vi "Get Terminal Refs for New Frame.vi"(8 "error in (no error)":errorcluster, 10 "Case Structure Ref":refnum<vi>, 11 "Setter Generator In":refnum<class "Setter Generator.lvclass">) -> (0 "error out":errorcluster, 2 "reference out":refnum<vi>, 3 "Setter Generator Out":refnum<class "Setter Generator.lvclass">)   [LabVIEW 2020, in "Method Generation.lvlib" / "Setter Generator.lvclass"]
uses:
  Setter Generator.lvclass
  Setter Generator.lvclass/Setter Generator.ctl
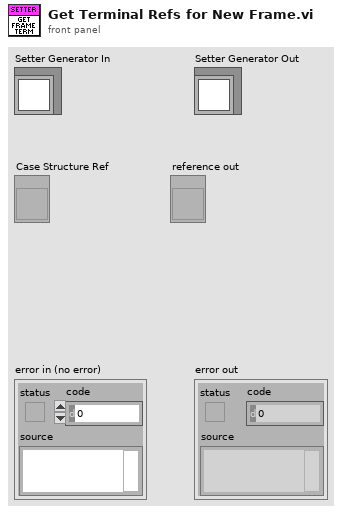
[diagram p1: front panel]
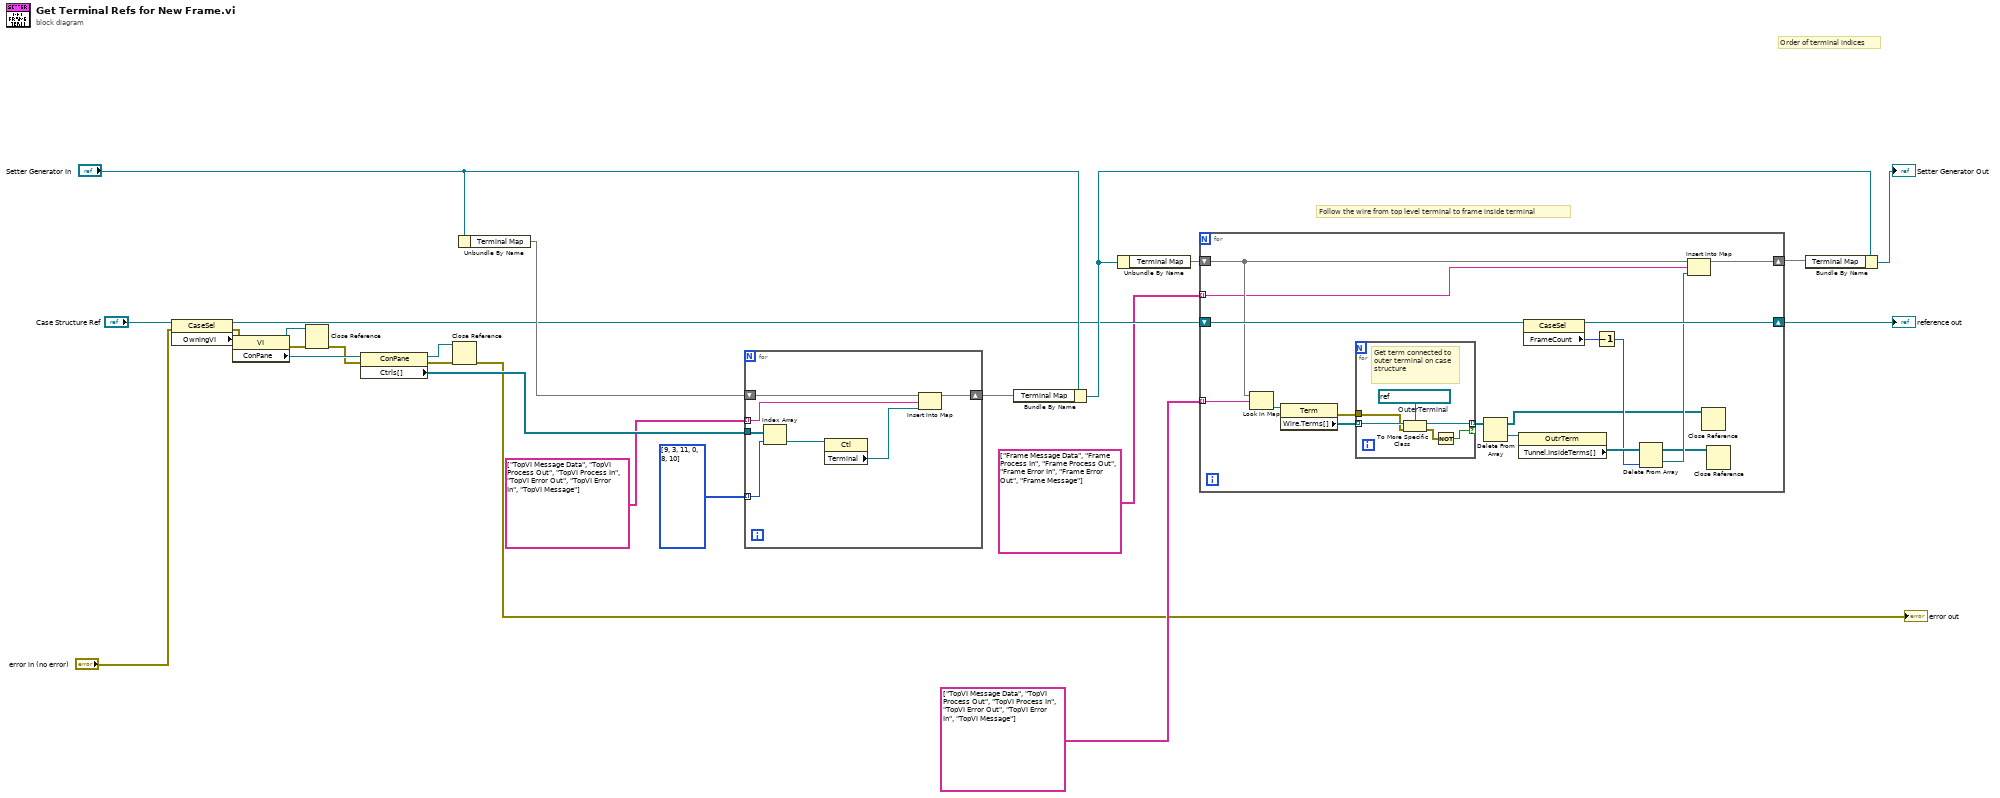
[diagram p0: block diagram]
diagram:
  # "Follow the wire from top level terminal to frame inside terminal"
  # "Order of terminal indices"
  n1 = property class="CaseSel"(reference="Case Structure Ref", error in="error in (no error)") -> (reference out=w15:refnum<vi>, error out=w19:errorcluster, "OwningVI"=w25:refnum<vi>)
  n2 = property class="VI"(reference=w25, error in=w19) -> (reference out=w7:refnum<vi>, error out=w18:errorcluster, "ConPane"=w23:refnum<vi>)
  n3 = Close Reference(reference=w7, error in (no error)=w18) -> (error out=w8:errorcluster)
  n4 = property class="ConPane"(reference=w23, error in=w8) -> (reference out=w5:refnum<vi>, error out=w6:errorcluster, "Ctrls[]"=w24:refnum<vi>[])
  n5 = Close Reference(reference=w5, error in (no error)=w6) -> (error out=→"error out":errorcluster)
  n6 = Unbundle By Name("Setter Generator In") -> ("Terminal Map"=w20:map{string, refnum<vi>})
  n7 = for {
    tunnel: w24 -> [w30]
    shift-right: [w31] -> w10
    shift-left: w20 -> [w32]
    tunnel: i32[] [9, 3, 11, 0, 8, 10] ("index") -> [w29] mode=indexing
    tunnel: string[] ["TopVI Message Data", "TopVI Process Out", "TopVI Process In", "TopVI Error Out", "TopVI Error In", "TopVI Message"] ("Array") -> [w26] mode=indexing
    n8 = Index Array(array=w30, index=w29) -> (element=w28:refnum<vi>)
    n9 = property class="Ctl"(reference=w28) -> ("Terminal"=w27:refnum<vi>)  [unwired: 1 in, 2 out]
    n10 = Insert Into Map(map in=w32, key=w26, value=w27) -> (map out=w31:map{string, refnum<vi>})  [unwired: 2 out]
  }
  n11 = Bundle By Name(cluster="Setter Generator In", "Terminal Map"=w10) -> (w16:refnum<class "Setter Generator.lvclass">)
  n12 = Unbundle By Name(w16) -> ("Terminal Map"=w13:map{string, refnum<vi>})
  n13 = for {
    shift-right: [w40] -> w14
    shift-left: w15 -> [w43]
    shift-right: [w36] -> w11
    shift-left: w13 -> [w39]
    tunnel: string[] ["TopVI Message Data", "TopVI Process Out", "TopVI Process In", "TopVI Error Out", "TopVI Error In", "TopVI Message"] ("Array") -> [w38] mode=indexing
    tunnel: string[] ["Frame Message Data", "Frame Process In", "Frame Process Out", "Frame Error In", "Frame Error Out", "Frame Message"] -> [w37] mode=indexing
    n14 = Look In Map(map=w39, key=w38) -> (value=w49:refnum<vi>)  [unwired: 1 in, 1 out]
    n15 = property class="Term"(reference=w49) -> (error out=w47:errorcluster, "Wire.Terms[]"=w48:refnum<vi>[])  [unwired: 1 in, 1 out]
    n16 = for {
      tunnel: w48 -> [w55] mode=indexing
      tunnel: [w53] -> w46 mode=indexing if=w51
      tunnel: w47 -> [w50]
      w54 = refnum<vi> refnum  # OuterTerminal
      # "Get term connected to outer terminal on case structure"
      n17 = To More Specific Class(target class=w54, reference=w55, error in=w50) -> (specific class reference=w53:refnum<vi>, error out=w52:errorcluster)
      n18 = Not(x=w52) -> (.not. x?=w51:bool)
    }
    n19 = Delete From Array(array=w46) -> (deleted portion=w45:refnum<vi>, array with subset deleted=w33:refnum<vi>[])  [unwired: 2 in]
    n20 = property class="OutrTerm"(reference=w45) -> ("Tunnel.InsideTerms[]"=w44:refnum<vi>[])  [unwired: 1 in, 2 out]
    n21 = property class="CaseSel"(reference=w43) -> (reference out=w40:refnum<vi>, "FrameCount"=w42:i32)  [unwired: 1 in, 1 out]
    n22 = Decrement(x=w42) -> (x-1=w41:i32)
    n23 = Delete From Array(array=w44, index=w41) -> (deleted portion=w35:refnum<vi>, array with subset deleted=w34:refnum<vi>[])  [unwired: 1 in]
    n24 = Insert Into Map(map in=w39, key=w37, value=w35) -> (map out=w36:map{string, refnum<vi>})  [unwired: 2 out]
    n25 = Close Reference(reference=w33) -> ()  [unwired: 1 in, 1 out]
    n26 = Close Reference(reference=w34) -> ()  [unwired: 1 in, 1 out]
  }
  "reference out" <- w14
  n27 = Bundle By Name(cluster=w16, "Terminal Map"=w11) -> (→"Setter Generator Out":refnum<class "Setter Generator.lvclass">)
